vi "rm.server.get scalar inputs.vi"(8 "error in (no error)":errorcluster, 11 "Item Ref in":T3 format="%.0x") -> (0 "error out":errorcluster, 2 "resources":T1[](array[typedef]), 3 "Item Ref out":T3 format="%.0x")   [LabVIEW 2016]
uses:
  <vilib>/NI Veristand/Custom Device API/Custom Device Item Ref.ctl
  Shared/resource.ctl
  Shared/resource type.ctl
  <vilib>/NI Veristand/Custom Device API/Custom Device API.lvlib
  Shared/RM.Shared.lvlib
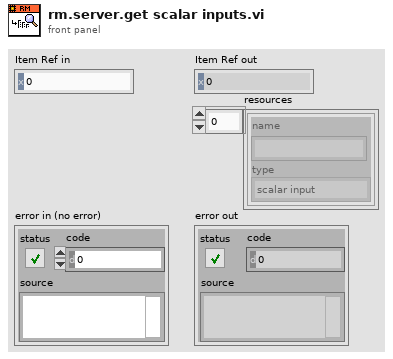
[diagram p1: front panel]
types:
  T1 = typedef "RM.Shared.lvlib/resource.ctl" = cluster{"name":string, "type":T2}
  T2 = typedef "resource type.ctl" = enum16{"scalar input", "scalar output", "waveform input", "waveform output"}
  T3 = typedef "Custom Device API.lvlib/Custom Device Item Ref.ctl" = u64
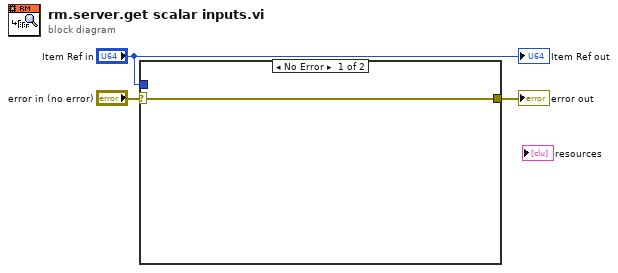
[diagram p0: block diagram]
diagram:
  n1 = case shown="No Error" "error in (no error)" {
    selector: "error in (no error)" -> [w4 w5]
    tunnel: [w4 w5] -> w2
    tunnel: "Item Ref in" -> [_ _]
    frame No Error {
    }
    frame Error {
    }
  }
  "error out" <- w2
  "Item Ref out" <- "Item Ref in"
